vi "AutoDetect Config Type.vi"(6 "overwrite type (F)":bool, 8 "error in (no error)":errorcluster, 11 "Attribute.Config in":refnum<class "Attribute.Config.lvclass">) -> (0 "error out":errorcluster, 3 "Attribute.Config out":refnum<class "Attribute.Config.lvclass">)   [LabVIEW 2013, in "Attribute.Config.lvclass"]
uses:
  Attribute.Config.lvclass
  Attribute.Config.lvclass/Attribute.Config.ctl
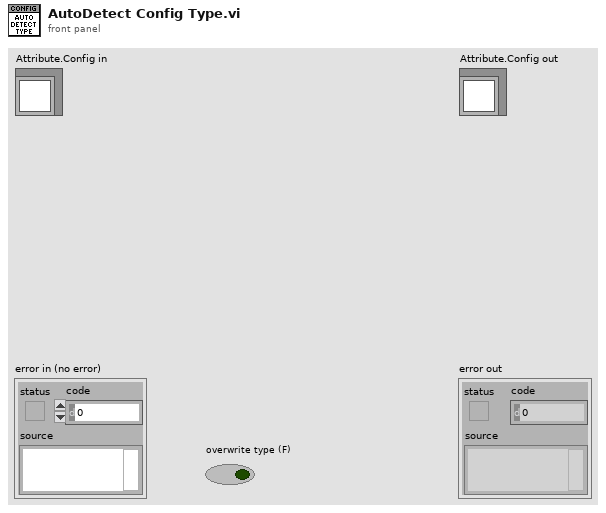
[diagram p1: front panel]
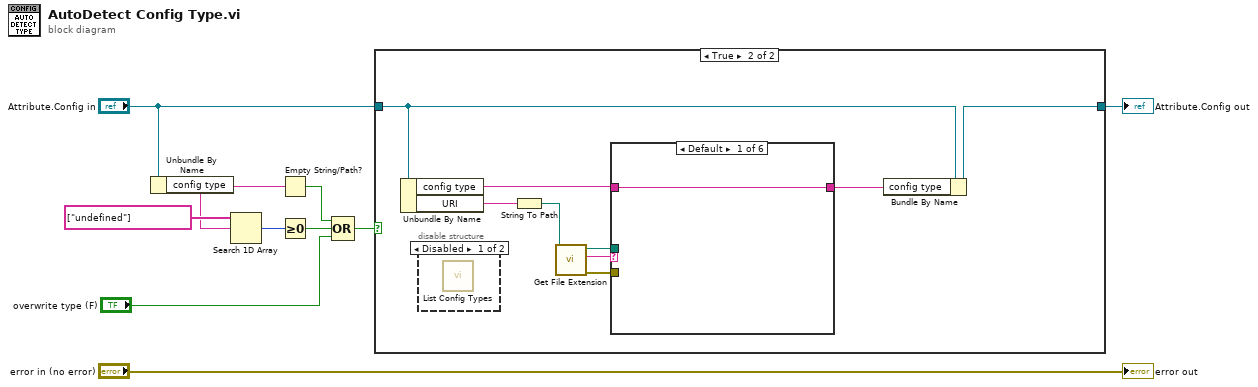
[diagram p0: block diagram]
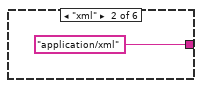
[diagram p4: hidden frame]
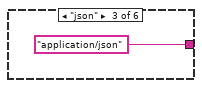
[diagram p5: hidden frame]
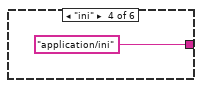
[diagram p6: hidden frame]
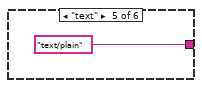
[diagram p7: hidden frame]
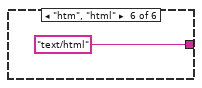
[diagram p8: hidden frame]
diagram:
  n1 = Unbundle By Name("Attribute.Config in") -> ("config type"=w4:string)
  n2 = Search 1D Array(1D array=string[] ["undefined"], element=w4) -> (index of element=w6:i32)  [unwired: 1 in]
  n3 = Empty String/Path?(string/path=w4) -> (empty?=w3:bool)
  n4 = Greater Or Equal To 0?(x=w6) -> (x >= 0?=w5:bool)
  n5 = Compound Arithmetic op=OR(w3, w5, "overwrite type (F)") -> (w1:bool)
  n6 = case shown="True" w1 {
    tunnel: "Attribute.Config in" -> [w11 w15]
    tunnel: [w11 w14] -> w8
    frame False {
    }
    frame True {
      n7 = Unbundle By Name(w15) -> ("config type"=w17:string, "URI"=w20:string)
      n8 = disable-structure shown="Disabled" {
        frame Disabled {
          n9 = call "List Config Types.vi"() -> ()  [unwired: 11 in, 1 out]
        }
        frame Enabled {
        }
      }
      n10 = String To Path(string=w20) -> (path=w19:path)
      n11 = call <vilib>:"Get File Extension.vi"("file"=w19) -> ("error out"=w13:errorcluster, "lowercase file extension"=w18:string, "dup file"=w12:path)  [unwired: 7 in, 1 out]
      n12 = case shown="Default" w18 {
        tunnel: w17 -> [w21 _ _ _ _ _]
        tunnel: [w21 "application/xml" ("config type") "application/json" ("config type") "application/ini" ("config type") "text/plain" ("config type") "text/html" ("config type")] -> w16
        tunnel: w13 -> [_ _ _ _ _ _]
        tunnel: w12 -> [_ _ _ _ _ _]
        frame Default {
        }
        frame "xml" {
        }
        frame "json" {
        }
        frame "ini" {
        }
        frame "text" {
        }
        frame "htm", "html" {
        }
      }
      n13 = Bundle By Name(cluster=w15, "config type"=w16) -> (w14:refnum<class "Attribute.Config.lvclass">)
    }
  }
  "Attribute.Config out" <- w8
  "error out" <- "error in (no error)"
